vi "Self Balancing Robot Main.vi"() -> ()   [LabVIEW 2014]
uses:
  <vilib>/myRIO/Instrument Drivers/Utilities/Utilities.lvlib
  <vilib>/myRIO/Instrument Drivers/Onboard IO/I2C/I2C.lvlib
  <vilib>/myRIO/Instrument Drivers/Onboard IO/I2C/typedefs/I2C Transfer Rate.ctl
  <vilib>/myRIO/Instrument Drivers/Onboard IO/I2C/typedefs/I2C User Configuration.ctl
  <vilib>/myRIO/Instrument Drivers/Onboard IO/DIO/DIO.lvlib
  <vilib>/platform/TimedLoop/XDataNode/XDataNode.xnode
  <vilib>/Platform/TimedLoop/XDataNode/nitl_modes.ctl
  <vilib>/Platform/TimedLoop/XDataNode/XDNodeRunTimeDep.lvlib
  <vilib>/Platform/TimedLoop/XDataNode/wakeup.ctl
  <vilib>/Platform/TimedLoop/XDataNode/timing_clust.ctl
  <vilib>/myRIO/Express VI/Onboard IO/DO/DO Express VI.xnode
  <vilib>/myRIO/Common/Instrument Driver Framework/myRIO v1.0/DIO/typedefs/DIO Channels Enum.ctl
  <vilib>/myRIO/Common/Instrument Driver Framework/myRIO v1.0/DIO/typedefs/DIO Channels List.ctl
  <vilib>/myRIO/Common/Instrument Driver Framework/Utilities/typedefs/Generic FPGA Reference.ctl
  <vilib>/myRIO/Common/Instrument Driver Framework/Utilities/typedefs/myRIO v1.0 Reference.ctl
  <vilib>/myRIO/Common/Instrument Driver Framework/Utilities/typedefs/Hardware Version Enum.ctl
  <vilib>/myRIO/Common/Instrument Driver Framework/Utilities/typedefs/myRIO Generic Hardware Reference.ctl
  <vilib>/myRIO/Instrument Drivers/Onboard IO/DIO/typedefs/DIO Reference.ctl
  <vilib>/myRIO/Instrument Drivers/Onboard IO/DIO/vis/myRIO DIO Open.xnode
  <vilib>/myRIO/Common/Instrument Driver Framework/Utilities/vis/Is FPGA Ref Available.vi
  <vilib>/myRIO/Instrument Drivers/Onboard Devices/Accelerometer/Accelerometer.lvlib
  <vilib>/myRIO/Common/Instrument Driver Framework/myRIO v1.0/DIO/vis/myRIO v1.1 Open DIO.vi
  <vilib>/userdefined/High Color/nirio_resource_hc.ctl
  <vilib>/myRIO/Express VI/Onboard IO/PWM/PWM Express VI.xnode
  <vilib>/myRIO/Instrument Drivers/Onboard IO/PWM/vis/Set Duty Cycle and Frequency.vi
  <vilib>/myRIO/Instrument Drivers/Onboard IO/PWM/PWM.lvlib
  <vilib>/myRIO/Instrument Drivers/Onboard IO/PWM/typedefs/PWM Configuration.ctl
  <vilib>/myRIO/Common/Instrument Driver Framework/myRIO v1.0/PWM/typedefs/PWM Channels Enum.ctl
  <vilib>/myRIO/Instrument Drivers/Onboard IO/PWM/typedefs/PWM Reference.ctl
  <vilib>/myRIO/Instrument Drivers/Onboard IO/PWM/vis/myRIO PWM Open.xnode
  <vilib>/myRIO/Common/Instrument Driver Framework/myRIO v1.0/PWM/vis/myRIO v1.1 Open PWM.vi
panel:
  in  "dt":dbl
  out "Loop Execution Time(ms)":u32
  in  "Filtered Angle Offset":dbl=0.24 format="%#_8g"
  in  "Gyro Offset":dbl=-36.0
  in  "Kd":dbl=0.106
  in  "Kp":dbl=0.8 format="%#_13g"
  in  "Filter Alpha":dbl=0.98 format="%#_13g"
  out "Motor Duty Cycle Output":dbl(graph)=-0.9506188969619731
  out "FilteredAngle":dbl(graph)=-88.15565348417263
  in  "[ESC]":bool
  # "Self Balancing Robot Demo"
  # "For help on troubleshooting this example as well as a brief description of how this example works \nvisit the help document under the My Computer section of the Project Viewer"
  # "PD Controller \nCoefficients"
  # "Gyro Scaling"
  # "Complementary Filter"
  # "OUT_X_L"
  # "OUT_X_H"
  # "OUT_Y_L"
  # "OUT_Y_H"
  # "OUT_Z_L"
  # "OUT_Z_H"
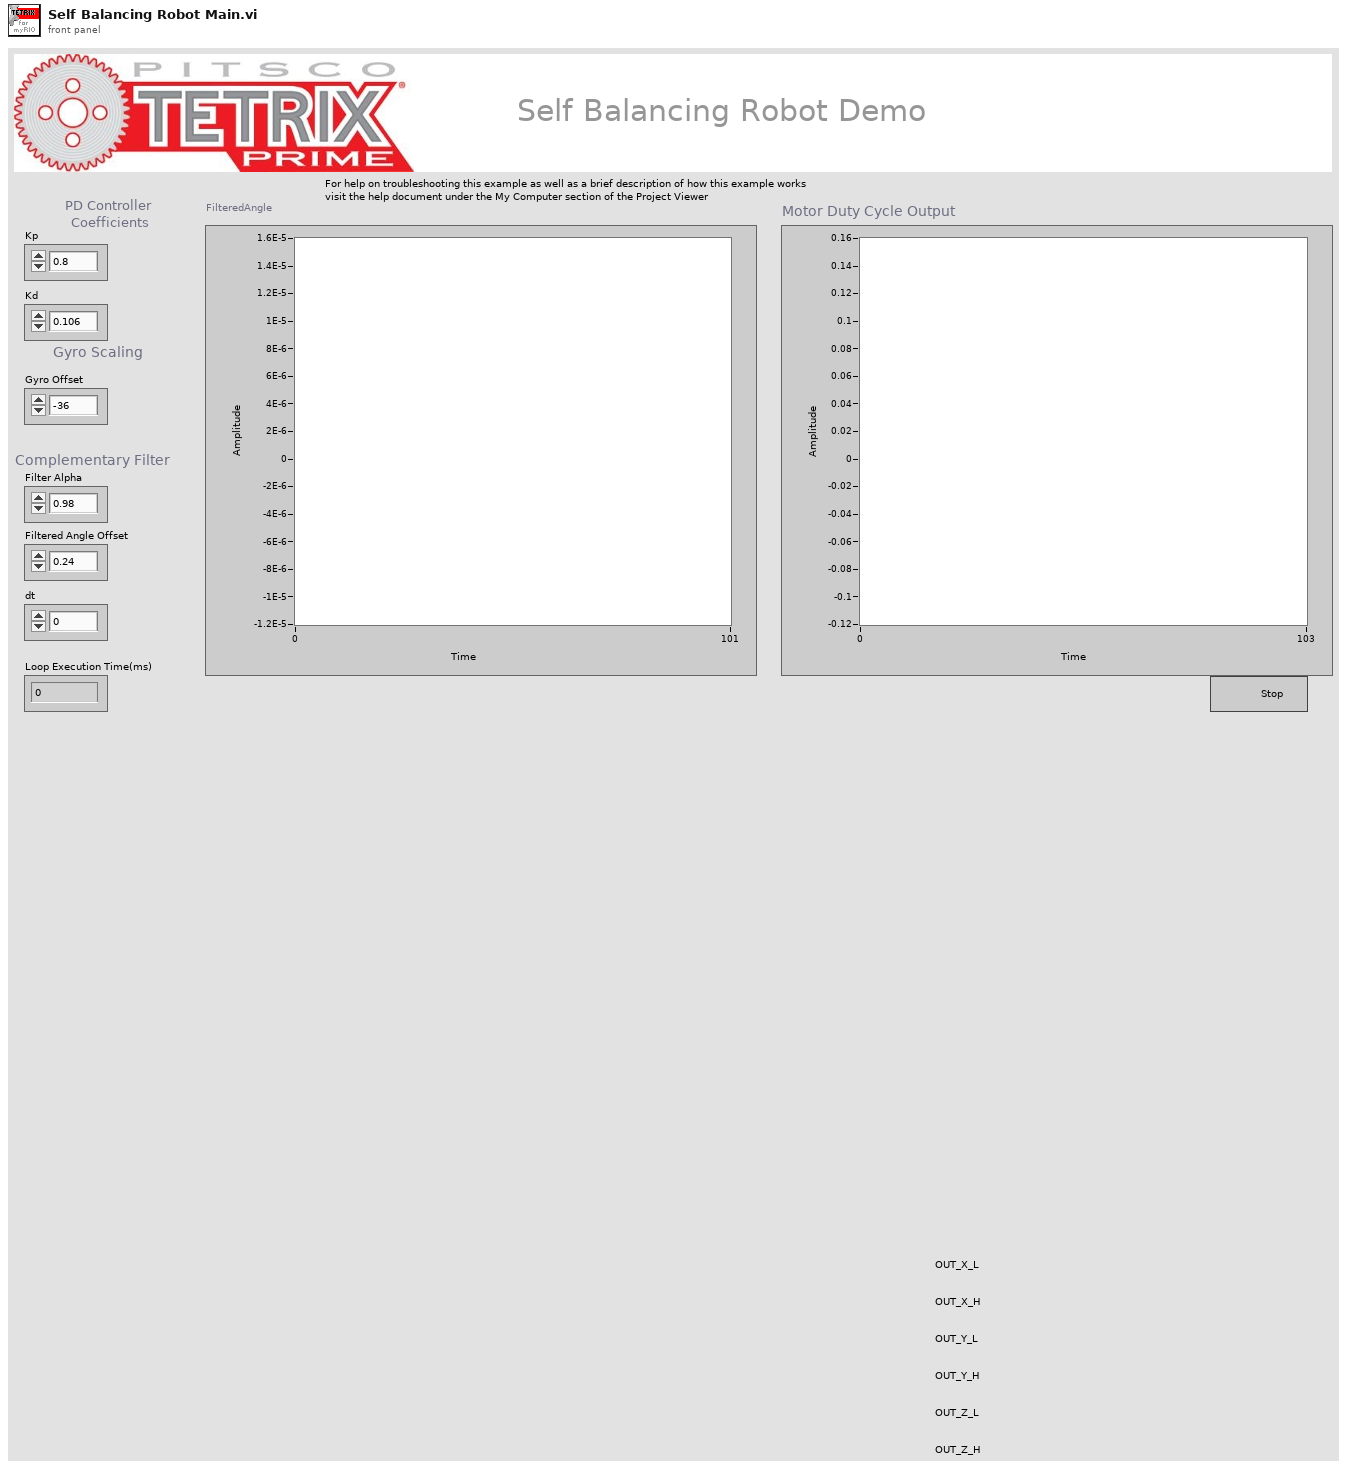
[diagram p1: front panel]
types:
  T1 = typedef "I2C.lvlib/I2C User Configuration.ctl" = cluster{"I2C Transfer Rate":T2}
  T2 = typedef "I2C.lvlib/I2C Transfer Rate.ctl" = enum16{"Standard mode (100 kbps)", "Fast mode (400 kbps)"}
  T3 = typedef "I2C.lvlib/I2C Reference.ctl" = cluster{"myRIO Reference":T4, "I2C Channels Enum":T8, "I2C Configuration":T9}
  T4 = typedef "myRIO Generic Hardware Reference.ctl" = cluster{"myRIO Model":T5, "myRIO Hardware Reference":T6}
  T5 = typedef "Hardware Version Enum.ctl" = enum16{"Unknown", "myRIO-1900", "myRIO-1950"}
  T6 = typedef "myRIO v1.0 Reference.ctl" = cluster{"Generic FPGA Reference":T7, "Allow multiple opens":bool}
  T7 = typedef "Generic FPGA Reference.ctl" = refnum<k20>
  T8 = typedef "I2C Channels Enum.ctl" = enum16{"Not Connected", "A/I2C", "B/I2C"}
  T9 = typedef "I2C.lvlib/I2C Configuration.ctl" = cluster{"I2C Transfer Rate":T2}
  T10 = typedef "Accelerometer.lvlib/Accelerometer Reference.ctl" = cluster{"myRIO Reference":T4, "Accelerometer Channels List":T11, "LSB Weight":dbl}
  T11 = typedef "Accelerometer Channels List.ctl" = T12[]
  T12 = typedef "Accelerometer Channels Enum.ctl" = enum16{"Not Connected", "X-Axis", "Y-Axis", "Z-Axis"}
  T13 = typedef "DIO.lvlib/DIO Reference.ctl" = cluster{"myRIO Reference":T4, "DIO Channels List":T14}
  T14 = typedef "DIO Channels List.ctl" = T15[]
  T15 = typedef "DIO Channels Enum.ctl" = enum16{"Not Connected", "C/DIO0", "C/DIO1", "C/DIO2", "C/DIO3", "C/DIO4", "C/DIO5", "C/DIO6", "C/DIO7", "A/DIO0", "A/DIO1", "A/DIO2", "A/DIO3", "A/DIO4", "A/DIO5", "A/DIO6", "A/DIO7", "A/DIO8", "A/DIO9", "A/DIO10", "A/DIO11", "A/DIO12", "A/DIO13", "A/DIO14", "A/DIO15", "B/DIO0", "B/DIO1", "B/DIO2", "B/DIO3", "B/DIO4", "B/DIO5", "B/DIO6", "B/DIO7", "B/DIO8", "B/DIO9", "B/DIO10", "B/DIO11", "B/DIO12", "B/DIO13", "B/DIO14", "B/DIO15", "LED0", "LED1", "LED2", "LED3", "Button0"}
  T16 = typedef "XDNodeRunTimeDep.lvlib/timing_clust.ctl" = cluster{"Expected End [f-1]":u64, "Actual End [f-1]":u64, "Finished Late? [f-1]":bool, "Expected End [i-1]":u64, "Actual End [i-1]":u64, "Finished Late? [i-1]":bool, "Expected Start [i]":u64, "Actual Start [i]":u64, "Expected Start [f]":u64, "Actual Start [f]":u64, "Source Name":string, "Structure Name":string, "Period":i64, "Deadline":i64, "Offset":i64, "Start":i64, "Priority":i32, "Timeout":i32, "Mode":T17, "Wakeup Reason":T18, "Error":errorcluster, "Source Type":string, "Secondary Source Type":string, "Global End Time":u64, "Global Start Time":u64, "Frame Duration":u64, "Iteration Duration":u64, "Assigned CPU":i32, "I/O Scan Engine Mode":u32}
  T17 = typedef "XDNodeRunTimeDep.lvlib/nitl_modes.ctl" = enum32{"No Change", "Process missed periods, maintain original phase", "Discard missed periods, maintain original phase", "Process missed periods, ignore original phase", "Discard missed periods, ignore original phase"}
  T18 = typedef "XDNodeRunTimeDep.lvlib/wakeup.ctl" = enum32{"Normal", "Aborted", "Asynchronous wakeup", "Timing source error", "Timed loop error", "Timeout"}
  T19 = typedef "PWM.lvlib/PWM Reference.ctl" = cluster{"myRIO Reference":T4, "PWM Channels Enum":T20, "PWM Configuration":T21}
  T20 = typedef "PWM Channels Enum.ctl" = enum16{"Not Connected", "C/PWM0", "C/PWM1", "A/PWM0", "A/PWM1", "A/PWM2", "B/PWM0", "B/PWM1", "B/PWM2"}
  T21 = typedef "PWM.lvlib/PWM Configuration.ctl" = cluster{"Frequency":dbl, "Duty Cycle":dbl}
  T22 = typedef "nirio_resource_hc.ctl" = tag
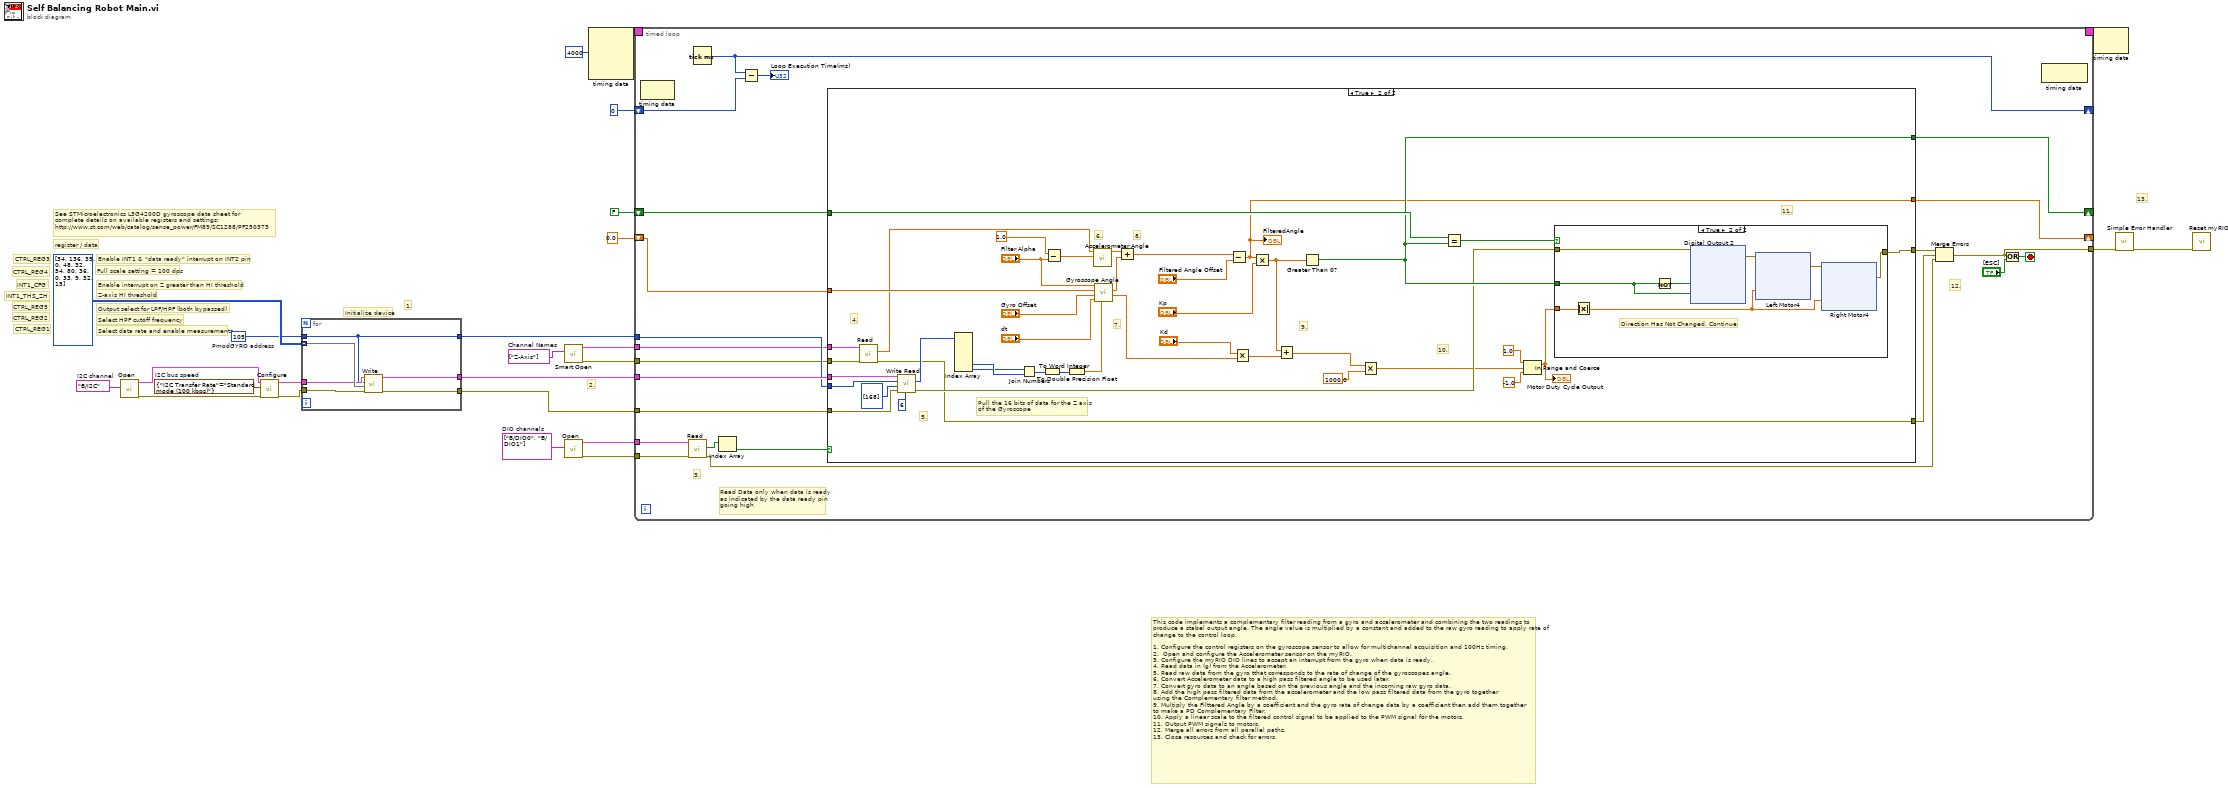
[diagram p0: block diagram]
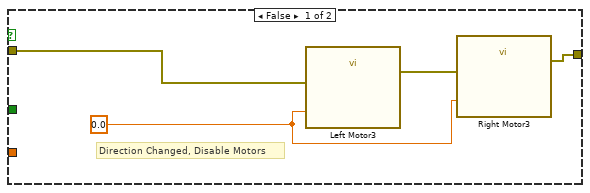
[diagram p3: hidden frame]
diagram:
  w5 = tag[] ["Z-Axis"]  # Channel Names
  w8 = tag[] ["B/DIO0", "B/DIO1"]  # DIO channels
  w20 = T1 {"I2C Transfer Rate"=enum."Standard mode (100 kbps)"}  # I2C bus speed
  w21 = tag "B/I2C"  # I2C channel
  w11 = u8 105  # PmodGYRO address
  # "This code implements a complementary filter reading from a gyro and accelerometer and combining the two readings to\nproduce a stabel output angle. The angle value is multiplied by a constant and added to the raw gyro reading to apply rate of\nchange to the control loop.\n \n1. Configure the control registers on the gyroscope sensor to allow for multichannel acquisition and 100Hz timing.\n2.  Open and configure the Accelerometer sensor on the myRIO.\n3. Configure the myRIO DIO lines to accept an interrupt from the gyro when data is ready.\n4. Read data in (g) from the Accelerometer.\n5. Read raw data from the gyro tthat corresponds to the rate of change of the gyroscopes angle.\n6. Convert Accelerometer data to a high pass filtered angle to be used later.\n7. Convert gyro data to an angle based on the previous angle and the incoming raw gyro data.\n8. Add the high pass filtered data from the accelerometer and the low pass filtered data from the gyro together\nusing the Complementary filter method.\n9. Multiply the Filttered Angle by a coefficient and the gyro rate of change data by a coefficient then add them together\nto make a PD Complementary Filter.\n10. Apply a linear scale to the filtered control signal to be applied to the PWM signal for the motors.\n11. Output PWM signals to motors.\n12. Merge all errors from all parallel paths.\n13. Close resources and check for errors."
  # "13."
  # "2."
  # "1."
  # "Enable INT1 & \"data ready\" interrupt on INT2 pin"
  # "CTRL_REG3"
  # "Select HPF cutoff frequency"
  # "CTRL_REG2"
  # "Output select for LPF/HPF (both bypassed)"
  # "CTRL_REG5"
  # "Initialize device"
  # "Select data rate and enable measurements"
  # "Z-axis HI threshold"
  # "Enable interrupt on Z greater than HI threshold"
  # "See STMicroelectronics L3G4200D gyroscope data sheet for\ncomplete details on available registers and settings:\nhttp://www.st.com/web/catalog/sense_power/FM89/SC1288/PF250373"
  # "CTRL_REG1"
  # "INT1_THS_ZH"
  # "INT1_CFG"
  # "Full scale setting = 100 dps"
  # "CTRL_REG4"
  # "register / data"
  n1 = call <vilib>:"Open.vi"("Channel Name"=w21) -> ("error out"=w18:errorcluster, "I2C Ref Out"=w19:T3)  [unwired: 9 in]
  n2 = call <vilib>:"Configure.vi"("error in (no error)"=w18, "I2C User Configuration"=w20, "I2C Ref In"=w19) -> ("error out"=w12:errorcluster, "I2C Ref Out"=w13:T3)  [unwired: 7 in]
  n3 = for {
    tunnel: [w31] -> w17
    tunnel: [w30] -> w16
    tunnel: [w26] -> w15
    tunnel: u8[][] [[34, 136], [35, 0], [48, 32], [54, 80], [36, 0], [33, 9], [32, 15]] ("Bytes to Write") -> [w29] mode=indexing
    tunnel: w13 -> [w28]
    tunnel: w12 -> [w27]
    tunnel: w11 -> [w26]
    n4 = call <vilib>:"Write.vi"("error in (no error)"=w27, "Bytes to Write"=w29, "Slave Address (7-bit)"=w26, "I2C Ref In"=w28) -> ("error out"=w31:errorcluster, "I2C Ref Out"=w30:T3)  [unwired: 6 in]
  }
  n5 = call <vilib>:"Smart Open.vi"("Channel Names"=w5) -> ("error out"=w3:errorcluster, "Accelerometer Ref Out"=w4:T10)  [unwired: 9 in]
  n6 = call <vilib>:"Open.vi"("Channel Names"=w8) -> ("error out"=w10:errorcluster, "DIO Ref Out"=w9:T13)  [unwired: 9 in]
  n7 = node-c288(i64 4000 ("Period")) -> (w25:T16)  [unwired: 3 in]
  n8 = timed-loop {
    tunnel: [w43] -> w22
    tunnel: w15 -> [w49]
    tunnel: w17 -> [w51]
    tunnel: w16 -> [w50]
    tunnel: w10 -> [w48]
    tunnel: w9 -> [w47]
    timing: w25 -> [_]
    timing-out: [_] -> w24
    shift-right: [w41] -> _
    shift-left: FALSE -> [w42]
    shift-right: [w39] -> _
    shift-left: 0.0 -> [w40]
    tunnel: w4 -> [w38]
    tunnel: w3 -> [w37]
    shift-right: [w34] -> _
    shift-left: u32 0 ("millisecond timer value") -> [w35]
    stop <- w53 stop-if-true
    # "3."
    # "12."
    # "Read Data only when data is ready\nas indicated by the data ready pin\ngoing high"
    n9 = node-c288() -> ()  [unwired: 1 in, 1 out]
    n10 = call <vilib>:"Read.vi"("error in (no error)"=w48, "DIO Ref In"=w47) -> ("error out"=w32:errorcluster, "Values"=w44:bool[])  [unwired: 7 in, 1 out]
    n11 = Tick Count (ms)() -> (millisecond timer value=w34:u32)
    n12 = Index Array "Index Array"(array=w44) -> (element=w45:bool)  [unwired: 1 in]
    n13 = Subtract(x=w34, y=w35) -> (x-y=→"Loop Execution Time(ms)":u32)
    n14 = case shown="True" w45 {
      tunnel: w51 -> [w59 w93]
      tunnel: w50 -> [_ w94]
      tunnel: w49 -> [_ w96]
      tunnel: [w59 w88] -> w46
      tunnel: w42 -> [w58 w91]
      tunnel: [w58 w90] -> w41
      tunnel: w40 -> [w57 w74]
      tunnel: [w57 w69] -> w39
      tunnel: w38 -> [_ w71]
      tunnel: w37 -> [w56 w72]
      tunnel: [w56 w68] -> w33
      frame False {
        # "INT2 (data ready) deasserted"
      }
      frame True {
        # "Pull the 16 bits of data for the Z axis\nof the Gyroscope"
        # "11."
        # "10."
        # "9."
        # "8."
        # "7."
        # "6."
        # "5."
        # "4."
        n15 = call <vilib>:"Read.vi"("error in (no error)"=w72, "Accelerometer Ref In"=w71) -> ("error out"=w68:errorcluster, "Values"=w73:dbl[])  [unwired: 7 in, 1 out]
        n16 = call <vilib>:"Write Read.vi"("Byte Count"=u32 6, "error in (no error)"=w93, "Bytes to Write"=u8[] [168], "Slave Address (7-bit)"=w96, "I2C Ref In"=w94) -> ("error out"=w89:errorcluster, "Bytes Read"=w95:u8[])  [unwired: 3 in, 1 out]
        n17 = Index Array "Index Array"(array=w95) -> (element #5=w100:u8, element #6=w99:u8)  [unwired: 6 in, 4 out]
        n18 = Join Numbers(hi=w99, lo=w100) -> ((hi.lo)=w101:u16)
        n19 = To Word Integer(number=w101) -> (16bit integer=w77:i16)
        n20 = Subtract(x=1.0, y="Filter Alpha") -> (x-y=w65:dbl)
        n21 = To Double Precision Float(number=w77) -> (double precision float=w76:dbl)
        n22 = call "Accelerometer Angle.vi"("angle LPF"=w65, "Values"=w73) -> ("Numeric"=w87:dbl)  [unwired: 9 in]
        n23 = call "Gyroscope Angle.vi"("Raw Gyro Data"=w76, "dt"="dt", "Gyro Offset"="Gyro Offset", "Previous Filtered Angle"=w74, "angle HPF"="Filter Alpha") -> ("Gyro Angle Rate"=w60:dbl, "Gyro Filtered Angle"=w86:dbl)  [unwired: 4 in, 1 out]
        n24 = Add(x=w87, y=w86) -> (x+y=w70:dbl)
        n25 = Subtract(x=w70, y="Filtered Angle Offset") -> (x-y=w69:dbl)
        "FilteredAngle" <- w69
        n26 = Multiply(x="Kd", y=w60) -> (x*y=w83:dbl)
        n27 = Multiply(x=w69, y="Kp") -> (x*y=w79:dbl)
        n28 = Add(x=w79, y=w83) -> (x+y=w78:dbl)
        n29 = Greater Than 0?(x=w79) -> (x > 0?=w90:bool)
        n30 = Multiply(x=w78, y=1000.0) -> (x*y=w67:dbl)
        n31 = Equal?(x=w91, y=w90) -> (x = y?=w92:bool)
        n32 = In Range and Coerce(upper limit=1.0, x=w67, lower limit=-1.0) -> (coerced(x)=w80:dbl)  [unwired: 1 out]
        "Motor Duty Cycle Output" <- w80
        n33 = case shown="True" w92 {
          tunnel: w80 -> [_ w111]
          tunnel: [w103 w110] -> w88
          tunnel: w90 -> [_ w106]
          tunnel: w89 -> [w102 w108]
          frame False {
            w104 = 0.0 ("Duty Cycle (0-1)")
            # "Direction Changed, Disable Motors"
            n34 = call "Left Motor3"("Duty Cycle (0-1)"=w104, "error in (no error)"=w102) -> ("error out"=w105:errorcluster)  [unwired: 25 in]
            n35 = call "Right Motor3"("Duty Cycle (0-1)"=w104, "error in (no error)"=w105) -> ("error out"=w103:errorcluster)  [unwired: 25 in]
          }
          frame True {
            # "Direction Has Not Changed, Continue"
            n36 = Absolute Value(x=w111) -> (abs(x)=w109:dbl)
            n37 = Not(x=w106) -> (.not. x?=w107:bool)
            n38 = xnode "Digital Output 2"("Left Motor (B/DIO2 (Pin 15))"=w107, "Right Motor (B/DIO3 (Pin 17))"=w106, "error in (no error)"=w108) -> ("error out"=w112:errorcluster)
            n39 = xnode "Left Motor4"("Duty Cycle"=w109, "error in (no error)"=w112) -> ("error out"=w113:errorcluster)
            n40 = xnode "Right Motor4"("Duty Cycle"=w109, "error in (no error)"=w113) -> ("error out"=w110:errorcluster)
          }
        }
      }
    }
    n41 = Merge Errors "Merge Errors"(w46, w33, w32) -> (w43:errorcluster)
    n42 = Or(x=w43, y="[ESC]") -> (x .or. y?=w53:bool)
    n43 = node-c288() -> ()  [unwired: 1 in, 1 out]
  }
  n44 = node-c288(w24) -> ()  [unwired: 1 out]
  n45 = call <vilib>:"Simple Error Handler.vi"("error in (no error)"=w22) -> ("error out"=w23:errorcluster)  [unwired: 4 in, 4 out]
  n46 = call <vilib>:"Reset myRIO.vi"("error in (no error)"=w23) -> ()  [unwired: 10 in, 1 out]
